vi "Channel Interface.vi"(8 "error in (no error)":errorcluster, 11 "Node Ptr":T1 format="%.0x") -> (0 "error out":errorcluster)   [LabVIEW 2019, in "SLSC-12201 DIO System Explorer.lvlib"]
uses:
  SLSC-12201 DIO System Explorer.lvlib
  <vilib>/NI VeriStand/Custom Device API/Custom Device Item Ref.ctl
  <vilib>/NI VeriStand/Custom Device API/Custom Device Channel Type.ctl
  Shared/Constants.vi
  <vilib>/NI VeriStand/Custom Device API/Get Item Property (String).vi
  <vilib>/NI VeriStand/Custom Device API/Custom Device API.lvlib
  Shared/SLSC-12201 DIO Shared.lvlib
panel:
  out "Access":i32(ring) items=["None", "Read Only", "Write Only", "Read/Write"]
  out "SLSC Information":string
  out "Default Value":dbl
  in  "Header":cluster{"Section Name":string}={"Section Name"="Custom Device Item Settings"}
  in  "Description":string
  out "Name":string
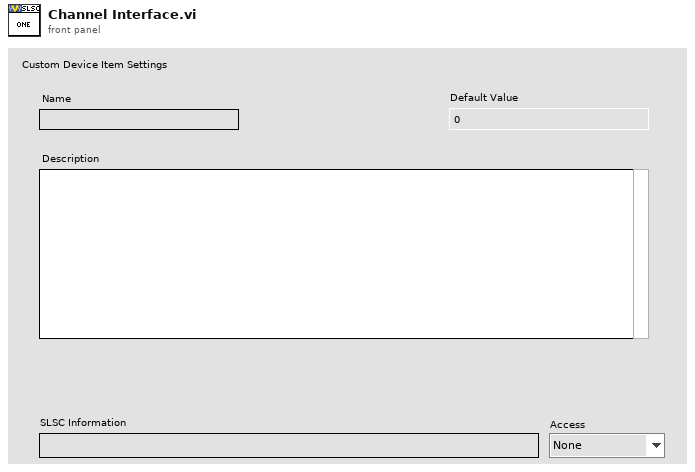
[diagram p1: front panel]
types:
  T1 = typedef "Custom Device API.lvlib/Custom Device Item Ref.ctl" = u64
  T2 = typedef "Custom Device API.lvlib/Custom Device Channel Type.ctl" = enum16{"Input", "Output"}
  T3 = typedef "Custom Device API.lvlib/Custom Device Item Info.ctl" = cluster{"Name":string, "Is Channel":bool, "GUID":string, "Is Waveform":bool}
  T4 = typedef "Custom Device API.lvlib/Custom Device Channel.ctl" = cluster{"Type":T2, "Units":string, "Default Value":dbl, "Faultable":bool, "Scalable":bool}
  T5 = typedef "Custom Device API.lvlib/Custom Device Commands.ctl" = enum16{"Default", "Item renamed", "Shutdown", "Dynamic button pressed"}
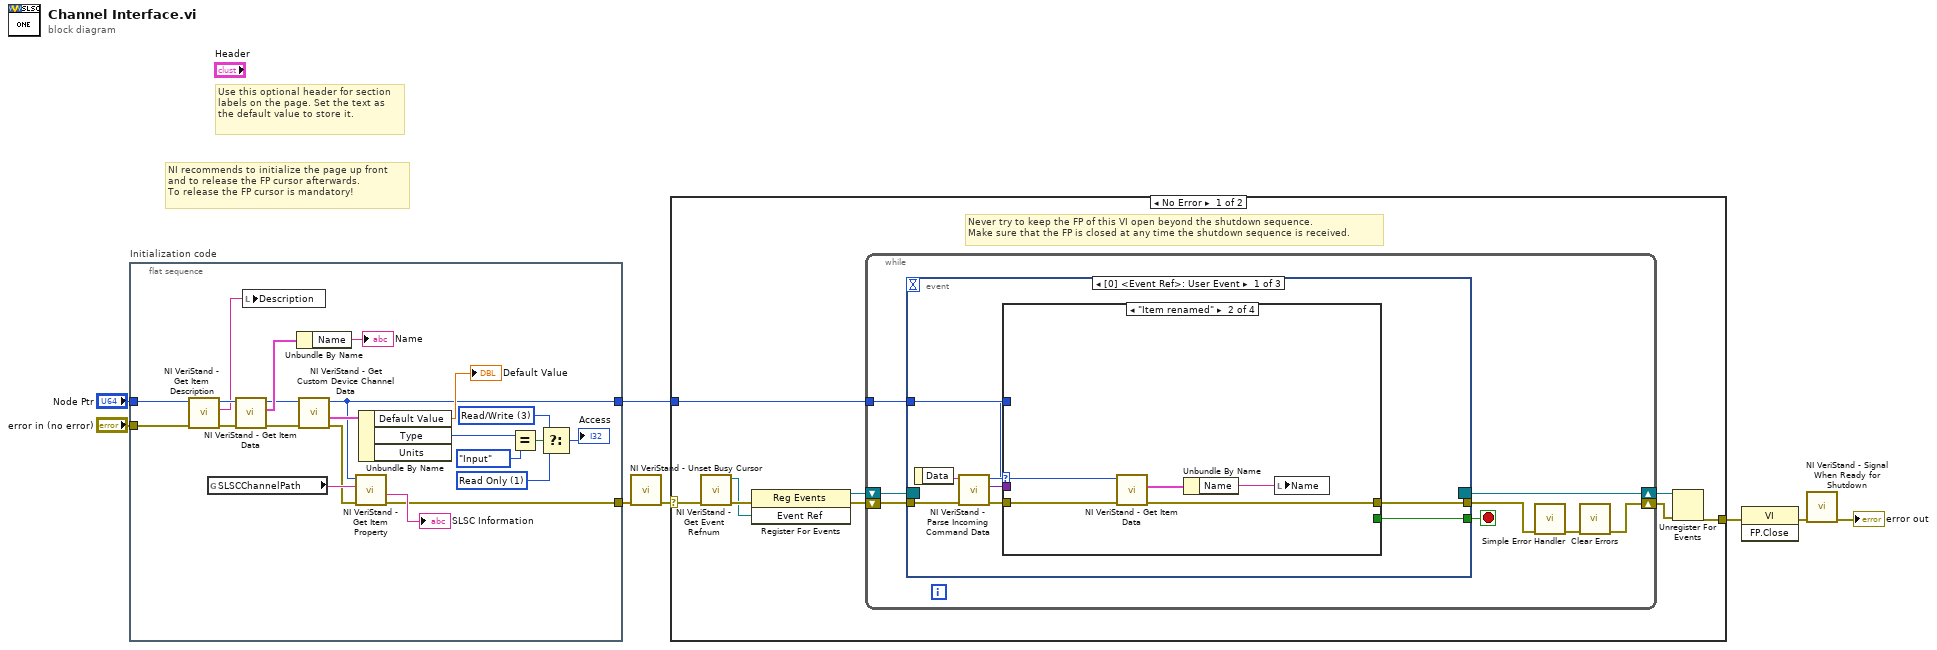
[diagram p0: block diagram]
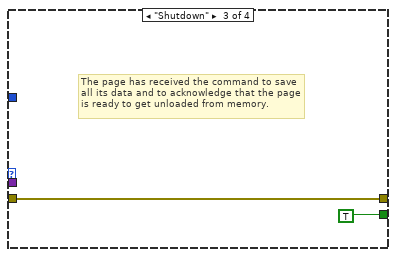
[diagram p3: hidden frame]
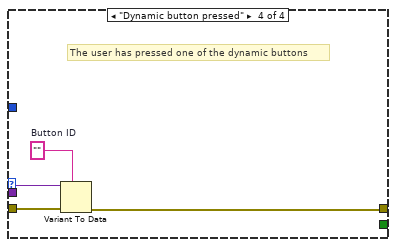
[diagram p4: hidden frame]
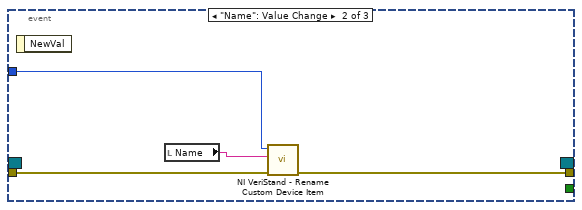
[diagram p5: hidden frame]
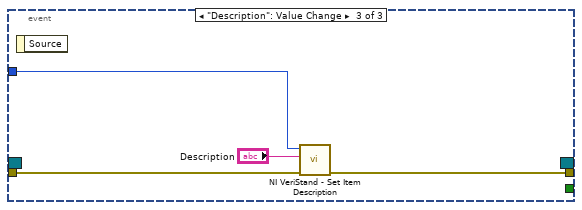
[diagram p6: hidden frame]
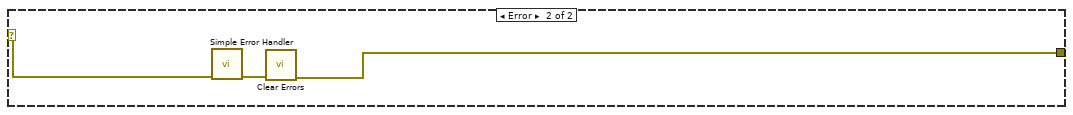
[diagram p7: hidden frame]
diagram:
  # "Use this optional header for section labels on the page. Set the text as the default value to store it."
  # "NI recommends to initialize the page up front\nand to release the FP cursor afterwards.\nTo release the FP cursor is mandatory!"
  n1 = flat-sequence "Initialization code" {
    tunnel: "error in (no error)" -> [w29]
    tunnel: "Node Ptr" -> [w28]
    tunnel: [w15] -> w4
    tunnel: [w18] -> w1
    frame #0 {
      w9 = 1 items=["None", "Read Only", "Write Only", "Read/Write"] ("Access")
      w10 = 3 items=["None", "Read Only", "Write Only", "Read/Write"] ("Access")
      n2 = call <vilib>:"NI VeriStand - Get Item Description.vi"("error in (no error)"=w29, "Item Ref in"=w28) -> ("error out"=w26:errorcluster, "Description"=w27:string, "Item Ref out"=w30:T1)  [unwired: 7 out]
      n3 = global read "Constants.vi" "SLSCChannelPath"() -> (w19:string)
      n4 = call <vilib>:"NI VeriStand - Get Item Data.vi"("error in (no error)"=w26, "Item Ref in"=w30) -> ("error out"=w22:errorcluster, "Item Info"=w25:T3, "Item Ref out"=w23:T1)  [unwired: 7 out]
      n5 = local write "Description"(w27) -> ()
      n6 = Unbundle By Name(w25) -> ("Name"=→"Name":string)
      n7 = call <vilib>:"NI VeriStand - Get Custom Device Channel Data.vi"("error in (no error)"=w22, "Channel Ref in"=w23) -> ("error out"=w16:errorcluster, "Channel"=w24:T4, "Channel Ref out"=w18:T1)  [unwired: 4 in, 3 out]
      n8 = call-poly <vilib>:"NI VeriStand - Get Item Property.vi"("error in (no error)"=w16, "Property Name"=w19, "Item Ref in"=w18) -> ("error out"=w15:errorcluster, "Value"=→"SLSC Information":string)  [unwired: 5 in, 2 out]
      n9 = Unbundle By Name(w24) -> ("Default Value"=→"Default Value":dbl, "Type"=w14:T2)  [unwired: 1 out]
      n10 = Equal?(x=w14, y=Custom_Device_Channel_Type."Input") -> (x = y?=w12:bool)
      n11 = Select(t=w10, s=w12, f=w9) -> (s? t:f=→"Access":i32)
    }
  }
  n12 = call <vilib>:"NI VeriStand - Unset Busy Cursor.vi"("error in (no error)"=w4) -> ("error out"=w3:errorcluster)  [unwired: 10 out]
  n13 = case shown="No Error" w3 {
    selector: w3 -> [w31 w78]
    tunnel: [w36 w76] -> w8
    tunnel: w1 -> [w32 _]
    frame No Error {
      # "Never try to keep the FP of this VI open beyond the shutdown sequence.\nMake sure that the FP is closed at any time the shutdown sequence is received."
      n14 = call <vilib>:"NI VeriStand - Get Event Refnum.vi"("error in (no error)"=w31) -> ("error out"=w39:errorcluster, "Event Ref"=w35:refnum<user-event>)  [unwired: 9 out]
      n15 = register-events(error in=w39, w35) -> (reference out=w33:refnum<event-registration>, error out=w34:errorcluster)  [unwired: 1 in]
      n16 = while {
        tunnel: w32 -> [w43]
        shift-right: [w40] -> w37
        shift-left: w34 -> [w46]
        shift-right: [w47] -> w38
        shift-left: w33 -> [w45]
        stop <- w44 stop-if-true
        n17 = event shown="[0] <Event Ref>: User Event" {
          selector: w45 -> [_ _ _]
          dyn-events: [_ _ _] -> w47
          timeout: _ -> [_ _ _]
          tunnel: w46 -> [w55 w71 w74]
          tunnel: [w51 _ _] -> w44
          tunnel: [w50 w70 w73] -> w42
          tunnel: w43 -> [w49 w69 w75]
          event User Event {
            n18 = event-data() -> ("Data"=w54:string)  [unwired: 1 out]
            n19 = call <vilib>:"NI VeriStand - Parse Incoming Command Data.vi"("error in (no error)"=w55, "Incoming data"=w54) -> ("error out"=w53:errorcluster, "Outgoing data"=w48:variant, "Action"=w52:T5)  [unwired: 7 out]
            n20 = case shown="\"Item renamed\"" w52 {
              tunnel: w53 -> [w56 w61 w62 w67]
              tunnel: [_ _ TRUE _] -> w51
              tunnel: [w56 w58 w62 w64] -> w50
              tunnel: w49 -> [_ w60 _ _]
              tunnel: w48 -> [_ _ _ w66]
              frame "Default", Default {
              }
              frame "Item renamed" {
                n21 = call <vilib>:"NI VeriStand - Get Item Data.vi"("error in (no error)"=w61, "Item Ref in"=w60) -> ("error out"=w58:errorcluster, "Item Info"=w59:T3)  [unwired: 8 out]
                n22 = Unbundle By Name(w59) -> ("Name"=w57:string)
                n23 = local write "Name"(w57) -> ()
              }
              frame "Shutdown" {
                # "The page has received the command to save all its data and to acknowledge that the page is ready to get unloaded from memory."
              }
              frame "Dynamic button pressed" {
                w65 = ""  # Button ID
                # "The user has pressed one of the dynamic buttons"
                n24 = Variant To Data(error in=w67, type=w65, Variant=w66) -> (error out=w64:errorcluster)  [unwired: 1 out]
              }
            }
          }
          event "Name": Value Change {
            n25 = event-data() -> ()  [unwired: 2 out]
            n26 = local read "Name"() -> (w68:string)
            n27 = call <vilib>:"NI VeriStand - Rename Custom Device Item.vi"("error in (no error)"=w71, "New Name"=w68, "Item Ref in"=w69) -> ("error out"=w70:errorcluster)  [unwired: 1 in, 7 out]
          }
          event "Description": Value Change {
            n28 = event-data() -> ()  [unwired: 2 out]
            n29 = call <vilib>:"NI VeriStand - Set Item Description.vi"("error in (no error)"=w74, "Description"="Description", "Item Ref in"=w75) -> ("error out"=w73:errorcluster)  [unwired: 8 out]
          }
        }
        n30 = call <vilib>:"Simple Error Handler.vi"("error in (no error)"=w42) -> ("error out"=w41:errorcluster)  [unwired: 1 in, 7 out]
        n31 = call <vilib>:"Clear Errors.vi"("error in (no error)"=w41) -> ("error out"=w40:errorcluster)  [unwired: 1 in, 5 out]
      }
      n32 = Unregister For Events(event registration refnum=w38, error in=w37) -> (error out=w36:errorcluster)
    }
    frame Error {
      n33 = call <vilib>:"Simple Error Handler.vi"("error in (no error)"=w78) -> ("error out"=w77:errorcluster)  [unwired: 1 in, 7 out]
      n34 = call <vilib>:"Clear Errors.vi"("error in (no error)"=w77) -> ("error out"=w76:errorcluster)  [unwired: 1 in, 5 out]
    }
  }
  n35 = invoke class="VI" method="FP.Close"(error in=w8) -> (error out=w7:errorcluster)  [unwired: 2 in, 2 out]
  n36 = call <vilib>:"NI VeriStand - Signal When Ready for Shutdown.vi"("error in (no error)"=w7) -> ("error out"=→"error out":errorcluster)  [unwired: 10 out]
